vi "Close.vi"(8 "Error In":errorcluster, 11 "SDO Manager":refnum<class "SDO Manager.lvclass">) -> (0 "Error Out":errorcluster, 3 "SDO Manager":refnum<class "SDO Manager.lvclass">)   [LabVIEW 2020, in "CANopen.lvlib" / "SDO Manager.lvlib" / "SDO Manager.lvclass"]
uses:
  SDO Manager.lvclass
  SDO Manager.lvclass/SDO Manager.ctl
  <vilib>/ActorFramework/Stop Msg/Stop Msg.lvclass
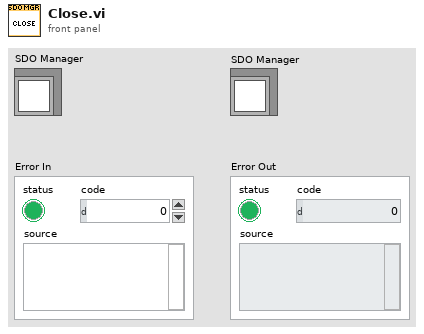
[diagram p1: front panel]
types:
  T1 = typedef "Semaphore RefNum" = refnum<k1>
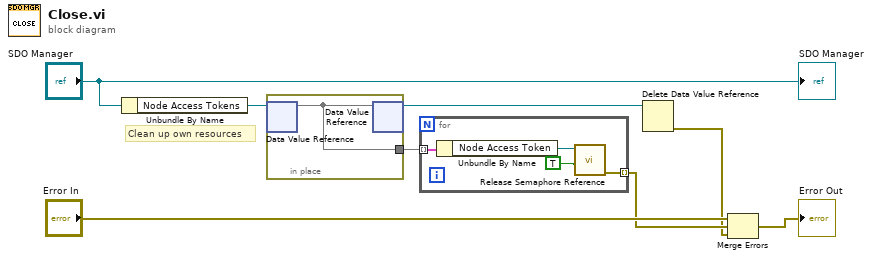
[diagram p0: block diagram]
diagram:
  # "Clean up own resources"
  n1 = Unbundle By Name("SDO Manager") -> ("Node Access Tokens"=w6:refnum<data-value>)
  n2 = in-place {
    in-place-border: [w9] -> w5
    n3 = in-place-dvr #1(w6) -> (w9:map{u8, T1})  [unwired: 1 out]
    n4 = in-place-dvr #1(w9) -> (w4:refnum<data-value>)  [unwired: 1 out]
  }
  n5 = for {
    tunnel: w5 -> [w13] mode=indexing
    tunnel: [w10] -> w2 mode=indexing
    n6 = Unbundle By Name(w13) -> ("Node Access Token"=w12:T1)
    n7 = call <vilib>:"Release Semaphore Reference.vi"("force destroy? (F)"=TRUE, "semaphore"=w12) -> ("error out"=w10:errorcluster)  [unwired: 8 in, 1 out]
  }
  n8 = Delete Data Value Reference(data value reference=w4) -> (error out=w1:errorcluster)  [unwired: 1 in, 1 out]
  n9 = Merge Errors("Error In", w2, w1) -> (→"Error Out":errorcluster)
  "SDO Manager" <- "SDO Manager"
